vi "Update Test-Assertion KVP.vi"(8 "error in (no error)":errorcluster, 10 "KVP":refnum<class "TestManagerMsg.KVP.lvclass">, 11 "Test Event Storage in":refnum<class "Test Event Storage.lvclass">) -> (0 "error out":errorcluster, 3 "Test Event Storage out":refnum<class "Test Event Storage.lvclass">)   [LabVIEW 2013, in "Caraya.lvlib" / "Test Event Storage.lvclass"]
uses:
  Test Event Storage.lvclass
  Test Manager Message KVP/TestManagerMsg.KVP.lvclass
  Test Event Storage.lvclass/Test Event Storage.ctl
  Test Result/Assert Event Data.ctl
  Test Manager Message/TestManagerMsg.lvclass/TestManagerMsg.ctl
  Test Manager Message KVP/TestManagerMsg.KVP.lvclass/TestManagerMsg.KVP.ctl
  assert store -- cluster.ctl
  Test Manager Message Assertion/TestManagerMsg.Assertion.lvclass
  Test Manager Message Verbose/TestManagerMsg.Verbose.lvclass
  test store -- cluster.ctl
  Test Manager Message Test/TestManagerMsg.Test.lvclass
  Test Manager Message/TestManagerMsg.lvclass
  Test Result/Test Result.lvclass
  Test Result/Test Registration Data.ctl
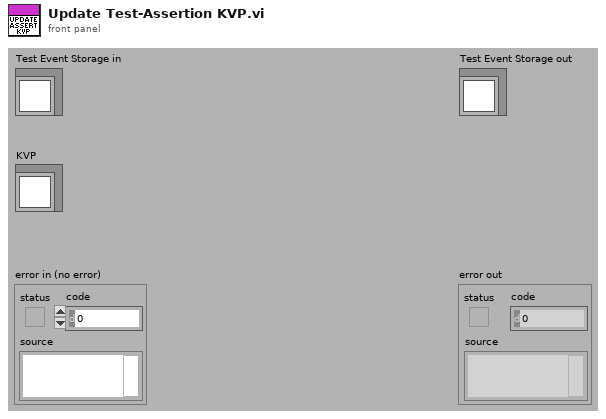
[diagram p1: front panel]
types:
  T1 = typedef "Caraya.lvlib/Test Result.lvclass/Assert Event Data.ctl" = cluster{"Name":string, "Passed":bool, "Call Chain":string[], "Test Error":errorcluster, "Time Stamp":timestamp, "Unique Assert ID":string, "Test ID":string, "Execution time (s)":dbl, "Verbose Explanation":string, "properties":variant, "measurements":variant, "limits":variant}
  T2 = typedef "Caraya.lvlib/Test Result.lvclass/Test Registration Data.ctl" = cluster{"Name":string, "Call Chain":string[], "Time Stamp":timestamp, "Test ID":string, "Caller ID":string}
  T3 = typedef "Caraya.lvlib/Test Event Storage.lvclass/assert store -- cluster.ctl" = cluster{"Assertion":refnum<class "TestManagerMsg.Assertion.lvclass">, "Explanation":refnum<class "TestManagerMsg.Verbose.lvclass">, "properties":variant, "measurements":variant, "limits":variant}
  T4 = typedef "Caraya.lvlib/Test Event Storage.lvclass/test store -- cluster.ctl" = cluster{"Test":refnum<class "TestManagerMsg.Test.lvclass">, "Defined":bool, "Passed":bool, "properties":variant, "assert-ids":variant}
  T5 = typedef "Caraya.lvlib/Test Event Storage.lvclass/store version -- enum.ctl" = enum16{"v1", "v2"}
  T6 = typedef "Caraya.lvlib/Test Event Storage.lvclass/Store Type -- enum.ctl" = enum16{"Suite", "Test", "Assert", "none"}
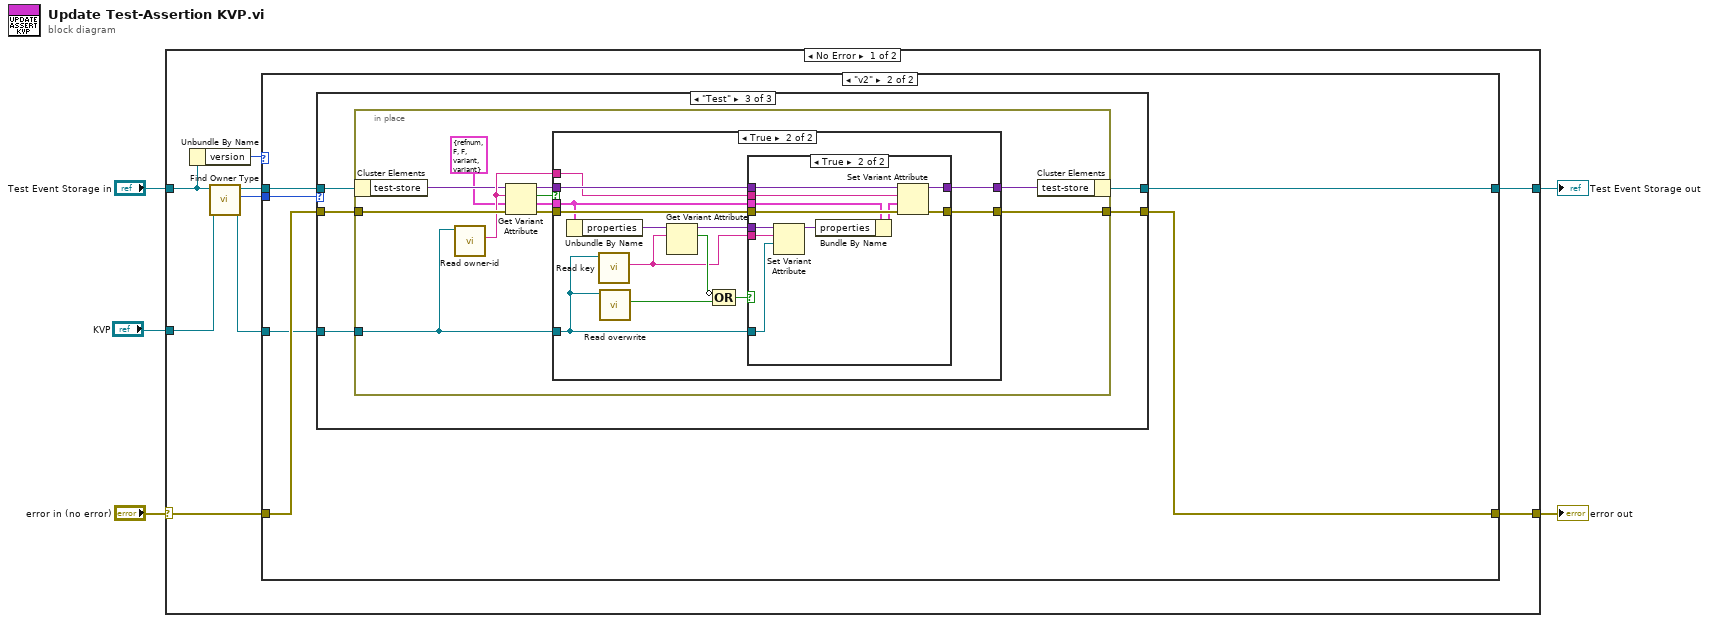
[diagram p0: block diagram]
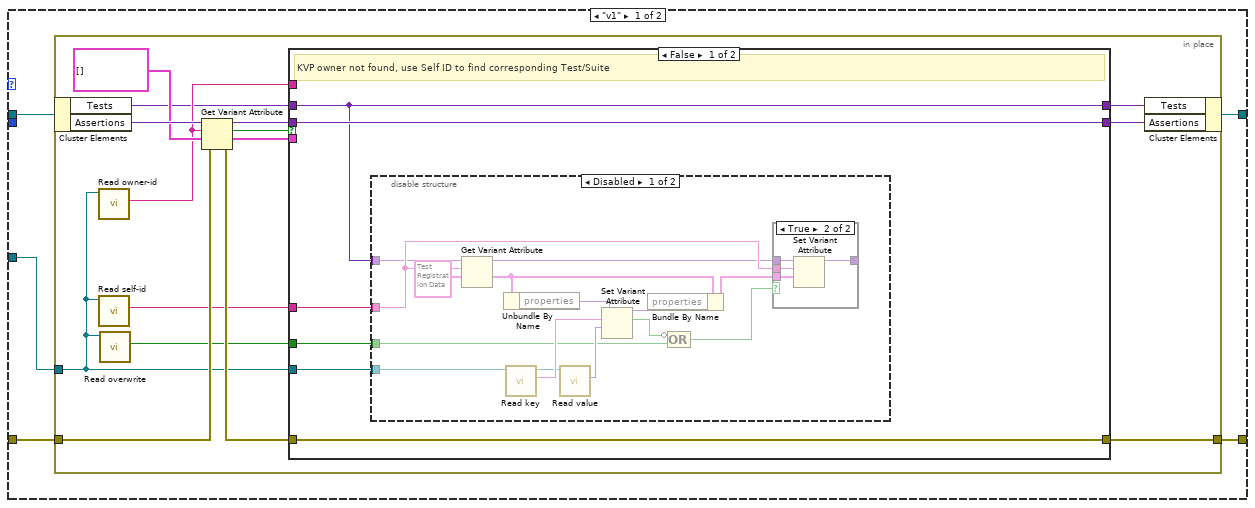
[diagram p2: hidden frame]
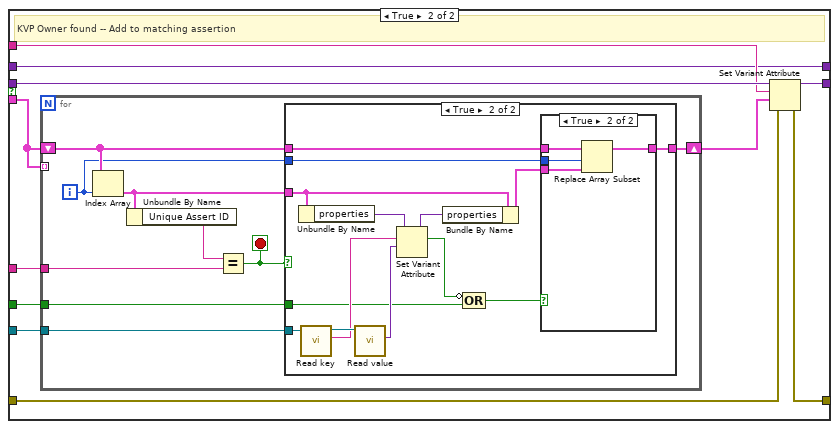
[diagram p5: hidden frame]
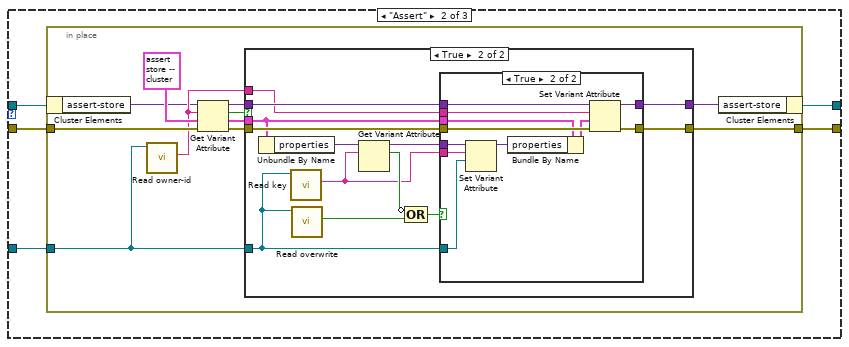
[diagram p9: hidden frame]
diagram:
  n1 = case shown="No Error" "error in (no error)" {
    selector: "error in (no error)" -> [w12 w198]
    tunnel: [w14 w198] -> w4
    tunnel: [w13 w197] -> w2
    tunnel: "Test Event Storage in" -> [w10 w197]
    tunnel: "KVP" -> [w7 _]
    frame No Error {
      n2 = Unbundle By Name(w10) -> ("version"=w11:T5)
      n3 = call "Find Owner Type.vi"("Message"=w7, "Test Event Storage in"=w10) -> ("Message dup"=w6:refnum<class "TestManagerMsg.KVP.lvclass">, "Owner Type"=w8:T6, "Test Event Storage out"=w9:refnum<class "Test Event Storage.lvclass">)  [unwired: 7 in]
      n4 = case shown="\"v2\"" w11 {
        tunnel: [w19 w102] -> w14
        tunnel: [w18 w103] -> w13
        tunnel: w12 -> [w17 w104]
        tunnel: w9 -> [w16 w105]
        tunnel: w8 -> [_ w106]
        tunnel: w6 -> [w15 w101]
        frame "v1" {
          n5 = in-place {
            in-place-border: w17 -> [w28]
            in-place-border: [w33] -> w19
            in-place-border: w15 -> [w22]
            n6 = in-place-cluster #1(w16) -> ("Tests"=w21:variant, "Assertions"=w31:variant)
            n7 = call "Read owner-id.vi"("TestManagerMsg in"=w22) -> ("owner-id"=w24:string)  [unwired: 9 in, 1 out]
            n8 = call "Read self-id.vi"("TestManagerMsg in"=w22) -> ("self-id"=w25:string)  [unwired: 9 in, 1 out]
            n9 = call "Read overwrite.vi"("TestManagerMsg in"=w22) -> ("overwrite?"=w23:bool)  [unwired: 9 in, 1 out]
            n10 = Get Variant Attribute(Variant=w31, name=w24, default value (empty Variant)=T1[] [] ("Assertions"), error in=w28) -> (duplicate Variant=w32:variant, found=w30:bool, value=w29:T1[], error out=w27:errorcluster)
            n11 = case shown="False" w30 {
              tunnel: [w40 w71] -> w34
              tunnel: [w39 w70] -> w33
              tunnel: w27 -> [w39 w69]
              tunnel: w32 -> [w40 w68]
              tunnel: w24 -> [_ w67]
              tunnel: w29 -> [_ w62]
              tunnel: w22 -> [w37 w66]
              tunnel: w25 -> [w36 w64]
              tunnel: w23 -> [w38 w63]
              tunnel: w21 -> [w35 w61]
              tunnel: [w35 w61] -> w20
              frame False {
                # "KVP owner not found, use Self ID to find corresponding Test/Suite"
                n12 = disable-structure shown="Disabled" {
                  disable-tunnel: w38 -> [w48 _]
                  disable-tunnel: w37 -> [w47 _]
                  disable-tunnel: w36 -> [w45 _]
                  disable-tunnel: w35 -> [w41 _]
                  frame Disabled {
                    n13 = Get Variant Attribute(Variant=w41, name=w45, default value (empty Variant)=T2 {"Name"="", "Call Chain"=[], "Time Stamp"=timestamp(0 s since 1904-01-01), "Test ID"="", "Caller ID"=""} ("Test Registration")) -> (duplicate Variant=w42:variant, value=w46:T2)  [unwired: 1 in, 2 out]
                    n14 = Unbundle By Name(w46) -> ("properties"=w50:variant)
                    n15 = call "Read key.vi"("TestManagerMsg in"=w47) -> ("key"=w52:string, "TestManagerMsg out"=w49:refnum<class "TestManagerMsg.KVP.lvclass">)  [unwired: 9 in]
                    n16 = call "Read value.vi"("TestManagerMsg.KVP in"=w49) -> ("value"=w51:variant)  [unwired: 9 in, 1 out]
                    n17 = Set Variant Attribute(Variant=w50, name=w52, value=w51) -> (Variant out=w53:variant, replaced=w54:bool)  [unwired: 1 in, 1 out]
                    n18 = Bundle By Name(cluster=w46, "properties"=w53) -> (w44:T2)
                    n19 = Compound Arithmetic op=OR(invert w54, w48) -> (w43:bool)
                    n20 = case shown="True" w43 {
                      tunnel: w42 -> [w56 w60]
                      tunnel: w45 -> [_ w59]
                      tunnel: w44 -> [_ w58]
                      tunnel: [w56 w57] -> _
                      frame False {
                      }
                      frame True {
                        n21 = Set Variant Attribute(Variant=w60, name=w59, value=w58) -> (Variant out=w57:variant)  [unwired: 1 in, 2 out]
                      }
                    }
                  }
                  frame Enabled {
                  }
                }
              }
              frame True {
                # "KVP Owner found -- Add to matching assertion"
                n22 = for {
                  tunnel: w66 -> [w80]
                  tunnel: w64 -> [w78]
                  tunnel: w63 -> [w77]
                  shift-right: [w79] -> w65
                  shift-left: w62 -> [w74]
                  tunnel: w62 -> [_] mode=indexing
                  i -> [w73]
                  stop <- w76 stop-if-true
                  n23 = Index Array(array=w74, index=w73) -> (element=w72:T1)
                  n24 = Unbundle By Name(w72) -> ("Unique Assert ID"=w75:string)
                  n25 = Equal?(x=w75, y=w78) -> (x = y?=w76:bool)
                  n26 = case shown="True" w76 {
                    tunnel: w80 -> [_ w95]
                    tunnel: [w81 w92] -> w79
                    tunnel: w74 -> [w81 w93]
                    tunnel: w77 -> [_ w84]
                    tunnel: w73 -> [_ w91]
                    tunnel: w72 -> [_ w90]
                    frame False {
                    }
                    frame True {
                      n27 = Unbundle By Name(w90) -> ("properties"=w88:variant)
                      n28 = call "Read key.vi"("TestManagerMsg in"=w95) -> ("key"=w86:string, "TestManagerMsg out"=w94:refnum<class "TestManagerMsg.KVP.lvclass">)  [unwired: 9 in]
                      n29 = call "Read value.vi"("TestManagerMsg.KVP in"=w94) -> ("value"=w87:variant)  [unwired: 9 in, 1 out]
                      n30 = Set Variant Attribute(Variant=w88, name=w86, value=w87) -> (Variant out=w85:variant, replaced=w83:bool)  [unwired: 1 in, 1 out]
                      n31 = Bundle By Name(cluster=w90, "properties"=w85) -> (w89:T1)
                      n32 = Compound Arithmetic op=OR(invert w83, w84) -> (w82:bool)
                      n33 = case shown="True" w82 {
                        tunnel: w93 -> [w96 w100]
                        tunnel: [w96 w99] -> w92
                        tunnel: w91 -> [_ w98]
                        tunnel: w89 -> [_ w97]
                        frame False {
                        }
                        frame True {
                          n34 = Replace Array Subset(array=w100, new element=w97, index=w98) -> (w99:T1[])
                        }
                      }
                    }
                  }
                }
                n35 = Set Variant Attribute(Variant=w68, name=w67, value=w65, error in=w69) -> (Variant out=w71:variant, error out=w70:errorcluster)  [unwired: 1 out]
              }
            }
            n36 = in-place-cluster #1("Tests"=w20, "Assertions"=w34) -> (w18:refnum<class "Test Event Storage.lvclass">)
          }
        }
        frame "v2" {
          n37 = case shown="\"Test\"" w106 {
            tunnel: w101 -> [_ w113 w157]
            tunnel: w104 -> [w107 w112 w156]
            tunnel: [w107 w111 w155] -> w102
            tunnel: [w108 w110 w154] -> w103
            tunnel: w105 -> [w108 w109 w153]
            frame "Suite", "none" {
              # "Not supported for Suites yet."
            }
            frame "Assert" {
              n38 = in-place {
                in-place-border: w112 -> [w122]
                in-place-border: [w123] -> w111
                in-place-border: w113 -> [w121]
                n39 = in-place-cluster #2(w109) -> ("assert-store"=w114:variant)
                n40 = call "Read owner-id.vi"("TestManagerMsg in"=w121) -> ("owner-id"=w115:string)  [unwired: 9 in, 1 out]
                n41 = Get Variant Attribute(Variant=w114, name=w115, default value (empty Variant)=T3 {"Assertion"=refnum, "Explanation"=refnum, "properties"=variant, "measurements"=variant, "limits"=variant} ("assert-store"), error in=w122) -> (duplicate Variant=w120:variant, found=w119:bool, value=w118:T3, error out=w117:errorcluster)
                n42 = case shown="True" w119 {
                  tunnel: [w126 w139] -> w124
                  tunnel: [w125 w138] -> w123
                  tunnel: w117 -> [w125 w137]
                  tunnel: w120 -> [w126 w136]
                  tunnel: w115 -> [_ w135]
                  tunnel: w118 -> [_ w134]
                  tunnel: w121 -> [_ w131]
                  frame False {
                  }
                  frame True {
                    n43 = Unbundle By Name(w134) -> ("properties"=w132:variant)
                    n44 = call "Read key.vi"("TestManagerMsg in"=w131) -> ("key"=w127:string)  [unwired: 9 in, 1 out]
                    n45 = call "Read overwrite.vi"("TestManagerMsg in"=w131) -> ("overwrite?"=w129:bool)  [unwired: 9 in, 1 out]
                    n46 = Get Variant Attribute(Variant=w132, name=w127) -> (duplicate Variant=w128:variant, found=w130:bool)  [unwired: 2 in, 2 out]
                    n47 = Compound Arithmetic op=OR(invert w130, w129) -> (w133:bool)
                    n48 = case shown="True" w133 {
                      tunnel: [w141 w152] -> w139
                      tunnel: [w140 w151] -> w138
                      tunnel: w137 -> [w140 w150]
                      tunnel: w136 -> [w141 w149]
                      tunnel: w135 -> [_ w148]
                      tunnel: w134 -> [_ w147]
                      tunnel: w131 -> [_ w142]
                      tunnel: w128 -> [_ w144]
                      tunnel: w127 -> [_ w143]
                      frame False {
                      }
                      frame True {
                        n49 = Set Variant Attribute(Variant=w144, name=w143, value=w142) -> (Variant out=w145:variant)  [unwired: 1 in, 2 out]
                        n50 = Bundle By Name(cluster=w147, "properties"=w145) -> (w146:T3)
                        n51 = Set Variant Attribute(Variant=w149, name=w148, value=w146, error in=w150) -> (Variant out=w152:variant, error out=w151:errorcluster)  [unwired: 1 out]
                      }
                    }
                  }
                }
                n52 = in-place-cluster #2("assert-store"=w124) -> (w110:refnum<class "Test Event Storage.lvclass">)
              }
            }
            frame "Test" {
              n53 = in-place {
                in-place-border: w156 -> [w166]
                in-place-border: [w167] -> w155
                in-place-border: w157 -> [w165]
                n54 = in-place-cluster #3(w153) -> ("test-store"=w159:variant)
                n55 = call "Read owner-id.vi"("TestManagerMsg in"=w165) -> ("owner-id"=w160:string)  [unwired: 9 in, 1 out]
                n56 = Get Variant Attribute(Variant=w159, name=w160, default value (empty Variant)=T4 {"Test"=refnum, "Defined"=FALSE, "Passed"=FALSE, "properties"=variant, "assert-ids"=variant} ("test-store"), error in=w166) -> (duplicate Variant=w164:variant, found=w163:bool, value=w162:T4, error out=w161:errorcluster)
                n57 = case shown="True" w163 {
                  tunnel: [w170 w183] -> w168
                  tunnel: [w169 w182] -> w167
                  tunnel: w161 -> [w169 w181]
                  tunnel: w164 -> [w170 w180]
                  tunnel: w160 -> [_ w179]
                  tunnel: w162 -> [_ w178]
                  tunnel: w165 -> [_ w175]
                  frame False {
                  }
                  frame True {
                    n58 = Unbundle By Name(w178) -> ("properties"=w176:variant)
                    n59 = call "Read key.vi"("TestManagerMsg in"=w175) -> ("key"=w171:string)  [unwired: 9 in, 1 out]
                    n60 = call "Read overwrite.vi"("TestManagerMsg in"=w175) -> ("overwrite?"=w173:bool)  [unwired: 9 in, 1 out]
                    n61 = Get Variant Attribute(Variant=w176, name=w171) -> (duplicate Variant=w172:variant, found=w174:bool)  [unwired: 2 in, 2 out]
                    n62 = Compound Arithmetic op=OR(invert w174, w173) -> (w177:bool)
                    n63 = case shown="True" w177 {
                      tunnel: [w185 w196] -> w183
                      tunnel: [w184 w195] -> w182
                      tunnel: w181 -> [w184 w194]
                      tunnel: w180 -> [w185 w193]
                      tunnel: w179 -> [_ w192]
                      tunnel: w178 -> [_ w191]
                      tunnel: w175 -> [_ w186]
                      tunnel: w172 -> [_ w188]
                      tunnel: w171 -> [_ w187]
                      frame False {
                      }
                      frame True {
                        n64 = Set Variant Attribute(Variant=w188, name=w187, value=w186) -> (Variant out=w189:variant)  [unwired: 1 in, 2 out]
                        n65 = Bundle By Name(cluster=w191, "properties"=w189) -> (w190:T4)
                        n66 = Set Variant Attribute(Variant=w193, name=w192, value=w190, error in=w194) -> (Variant out=w196:variant, error out=w195:errorcluster)  [unwired: 1 out]
                      }
                    }
                  }
                }
                n67 = in-place-cluster #3("test-store"=w168) -> (w154:refnum<class "Test Event Storage.lvclass">)
              }
            }
          }
        }
      }
    }
    frame Error {
    }
  }
  "error out" <- w4
  "Test Event Storage out" <- w2
